vi "LDA_Mirror_Setup.vi"(1 "Simulate/Run":T1=enum."Run VI") -> (4 "Mirror Traverse":string)   [LabVIEW 2022 SP3]
uses:
  Controls/User_Specific_mode.ctl
  Globals/Constants_global.vi
  Collision_Detection/Triangles/EnFlo specific/Collision Detection global.vi
  Globals/Trav_pos_global.vi
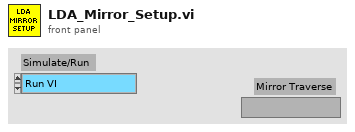
[diagram p1: front panel]
types:
  T1 = typedef "User_Specific_mode.ctl" = enum16{"Check VI only", "Run VI"}
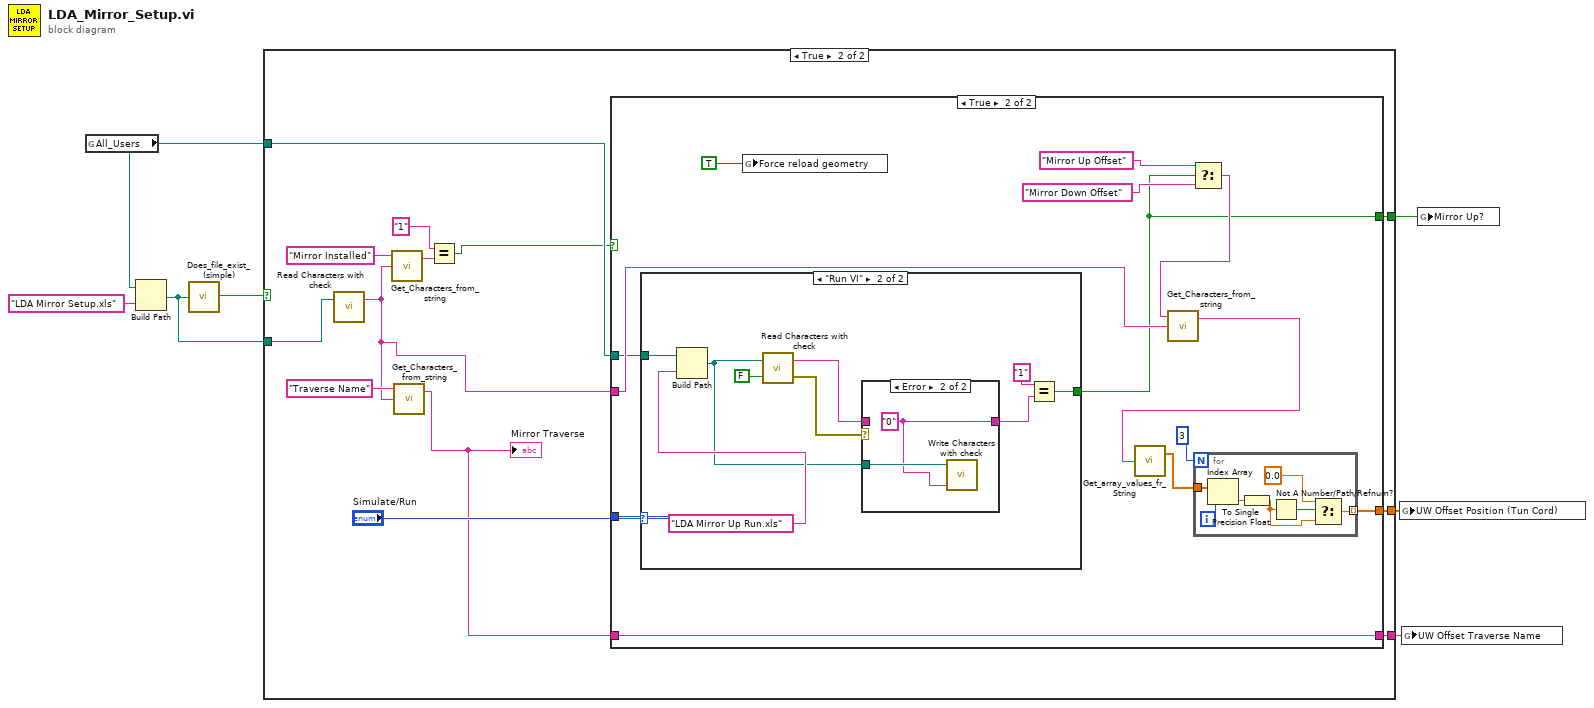
[diagram p0: block diagram]
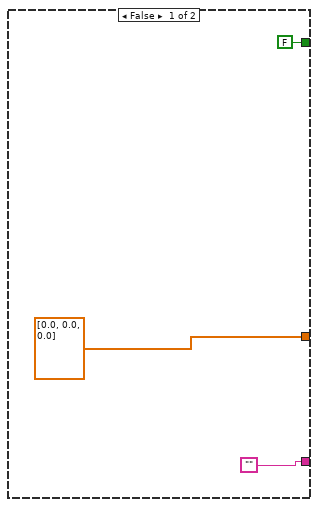
[diagram p2: hidden frame]
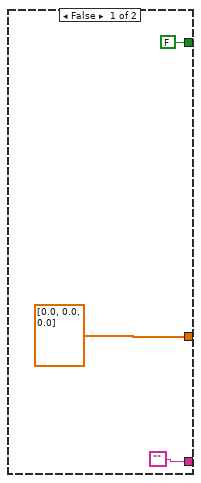
[diagram p3: hidden frame]
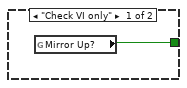
[diagram p4: hidden frame]
diagram:
  n1 = global read "Constants_global.vi" "All_Users"() -> (w6:path)
  n2 = Build Path(base path=w6, name or relative path="LDA Mirror Setup.xls") -> (appended path=w1:path)
  n3 = call "Does_file_exist_(simple).vi"("Pathname"=w1) -> ("exists?"=w2:bool)
  n4 = case shown="True" w2 {
    tunnel: w6 -> [_ w19]
    tunnel: [sgl[] [0.0, 0.0, 0.0] w17] -> w5
    tunnel: ["" w15] -> w4
    tunnel: [FALSE ("Mirror Up?") w13] -> w3
    tunnel: w1 -> [_ w11]
    frame False {
    }
    frame True {
      n5 = call "Read Characters with check.vi"("file (use dialog)"=w11) -> ("Read String"=w12:string)  [unwired: 1 in, 1 out]
      n6 = call "Get_Characters_from_string.vi"("Input string"=w12, "Variable name"="Mirror Installed") -> ("Value"=w21:string)  [unwired: 1 in, 1 out]
      n7 = call "Get_Characters_from_string.vi"("Input string"=w12, "Variable name"="Traverse Name") -> ("Value"=w14:string)  [unwired: 1 in, 1 out]
      "Mirror Traverse" <- w14
      n8 = Equal?(x="1" ("String to match"), y=w21) -> (x = y?=w16:bool)
      n9 = case shown="True" w16 {
        tunnel: [sgl[] [0.0, 0.0, 0.0] w33] -> w17
        tunnel: w19 -> [_ w29]
        tunnel: "Simulate/Run" -> [_ w28]
        tunnel: w12 -> [_ w32]
        tunnel: [FALSE w31] -> w13
        tunnel: ["" w30] -> w15
        tunnel: w14 -> [_ w30]
        frame False {
        }
        frame True {
          n10 = case shown="\"Run VI\"" w28 {
            tunnel: [w40 w47] -> w31
            tunnel: w29 -> [_ w46]
            frame "Check VI only" {
              n11 = global read "Trav_pos_global.vi" "Mirror Up?"() -> (w40:bool)
            }
            frame "Run VI" {
              n12 = Build Path(base path=w46, name or relative path="LDA Mirror Up Run.xls") -> (appended path=w44:path)
              n13 = call "Read Characters with check.vi"("Call EnFlo Error Handler?"=FALSE, "file (use dialog)"=w44) -> ("error out"=w42:errorcluster, "Read String"=w43:string)
              n14 = case shown="Error" w42 {
                tunnel: [w50 w51] -> w45
                tunnel: w43 -> [w50 _]
                tunnel: w44 -> [_ w52]
                frame No Error {
                }
                frame Error {
                  w51 = "0"
                  n15 = call "Write Characters with check.vi"("String to Write"=w51, "file (use dialog)"=w52) -> ()  [unwired: 2 in, 1 out]
                }
              }
              n16 = Equal?(x="1" ("String to match"), y=w45) -> (x = y?=w47:bool)
            }
          }
          n17 = global write "Collision Detection global.vi" "Force reload geometry"(TRUE ("Reload geometry")) -> ()
          n18 = Select(t="Mirror Up Offset", s=w31, f="Mirror Down Offset") -> (s? t:f=w37:string)
          n19 = call "Get_Characters_from_string.vi"("Input string"=w32, "Variable name"=w37) -> ("Value"=w34:string)  [unwired: 1 in, 1 out]
          n20 = call "Get_array_values_fr_String.vi"("String Value"=w34) -> ("Numeric Array"=w36:dbl[])  [unwired: 1 out]
          n21 = for {
            N: 3 -> [_]
            tunnel: [w59] -> w33 mode=indexing
            tunnel: w36 -> [w56]
            i -> [w55]
            n22 = Index Array(array=w56, index=w55) -> (element=w54:dbl)
            n23 = To Single Precision Float(number=w54) -> (single precision float=w53:sgl)
            n24 = Not A Number/Path/Refnum?(number/path/refnum=w53) -> (NaN/Path/Refnum?=w57:bool)
            n25 = Select(t=sgl 0.0, s=w57, f=w53) -> (s? t:f=w59:sgl)
          }
        }
      }
    }
  }
  n26 = global write "Trav_pos_global.vi" "UW Offset Position (Tun Cord)"(w5) -> ()
  n27 = global write "Trav_pos_global.vi" "UW Offset Traverse Name"(w4) -> ()
  n28 = global write "Trav_pos_global.vi" "Mirror Up?"(w3) -> ()
